vi "WriteConfig.vi"(8 "error in (no error)":errorcluster, 10 "Config":variant, 11 "RoomAlert in":refnum<class "RoomAlert.lvclass">) -> (0 "error out":errorcluster, 3 "RoomAlert out":refnum<class "RoomAlert.lvclass">)   [LabVIEW 2018, in "SensorPlugins.lvlib" / "RoomAlert.lvclass"]
doc: "Updates the configuration cluster."
uses:
  RoomAlert.lvclass
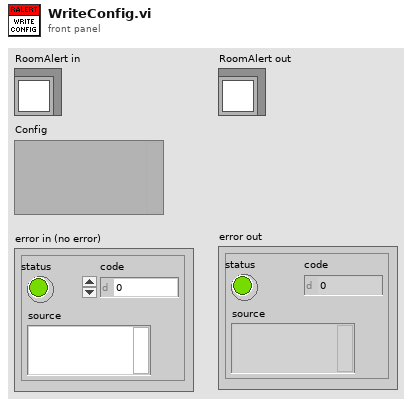
[diagram p1: front panel]
types:
  T1 = typedef "SensorPlugins.lvlib/RoomAlert.lvclass/MeasurementControls.ctl" = cluster{"Measurement RefreshTime (ms)":u32, "Measurement Name":string, "Timeout(ms)":i32, "Amber Warning Light Configuration":cluster{"Warning Temperture (Degrees C)":dbl, "Temperature Delta (Degrees C/Minute)":dbl, "Time Window (Minutes)":dbl}}
  T2 = typedef "SensorPlugins.lvlib/RoomAlert.lvclass/RoomAlertControls.ctl" = cluster{"Connected?":bool, "IP Address of SNMP Device":string, "Port (161)":u16, "Community Name":string, "Measurements To Read Array":u16[], "Update LightTower?":bool, "LightTower":cluster{"Red":bool, "Amber":bool, "Green":bool, "Audio":bool}, "RoomAlert Model ID":string, "Sensor OID Numbers":string[][], "Sensor Light Tower OID Numbers":string[][]}[]
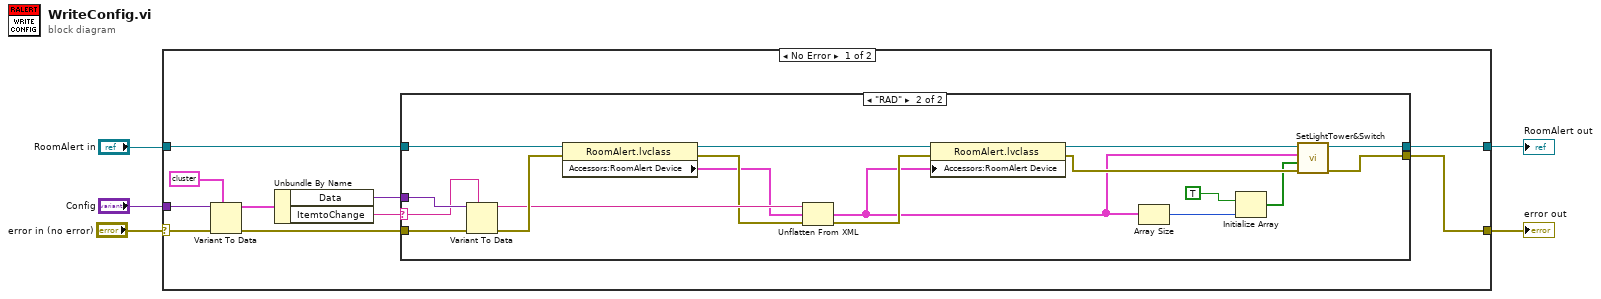
[diagram p0: block diagram]
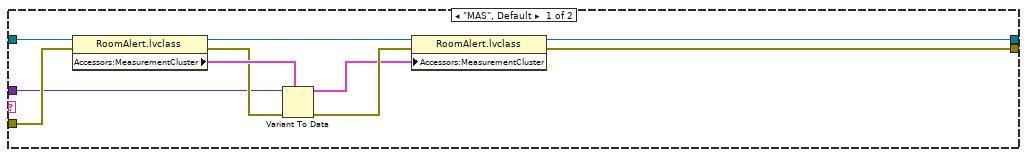
[diagram p2: hidden frame]
diagram:
  n1 = case shown="No Error" "error in (no error)" {
    selector: "error in (no error)" -> [w13 w45]
    tunnel: [w7 w45] -> w1
    tunnel: "RoomAlert in" -> [w15 w44]
    tunnel: [w6 w44] -> w2
    tunnel: "Config" -> [w14 _]
    frame No Error {
      n2 = Variant To Data(error in=w13, type=cluster{"Data":variant, "ItemtoChange":string} {"Data"=variant, "ItemtoChange"=""}, Variant=w14) -> (data=w10:cluster{"Data":variant, "ItemtoChange":string}, error out=w12:errorcluster)
      n3 = Unbundle By Name(w10) -> ("Data"=w9:variant, "ItemtoChange"=w8:string)
      n4 = case shown="\"RAD\"" w8 {
        selector: w8 -> [_ w38]
        tunnel: w15 -> [w25 w43]
        tunnel: [w23 w31] -> w6
        tunnel: [w22 w30] -> w7
        tunnel: w12 -> [w21 w40]
        tunnel: w9 -> [w18 w41]
        frame "MAS", Default {
          n5 = property class="RoomAlert.lvclass"(reference=w25, error in=w21) -> (reference out=w24:refnum<class "RoomAlert.lvclass">, error out=w19:errorcluster, "Accessors:MeasurementCluster"=w20:T1)
          n6 = Variant To Data(error in=w19, type=w20, Variant=w18) -> (data=w16:T1, error out=w17:errorcluster)
          n7 = property class="RoomAlert.lvclass"(reference=w24, error in=w17, "Accessors:MeasurementCluster"=w16) -> (reference out=w23:refnum<class "RoomAlert.lvclass">, error out=w22:errorcluster)
        }
        frame "RAD" {
          n8 = Variant To Data(error in=w40, type=w38, Variant=w41) -> (data=w37:string, error out=w39:errorcluster)
          n9 = property class="RoomAlert.lvclass"(reference=w43, error in=w39) -> (reference out=w42:refnum<class "RoomAlert.lvclass">, error out=w36:errorcluster, "Accessors:RoomAlert Device"=w35:T2)
          n10 = Unflatten From XML(xml string=w37, type=w35, error in (no error)=w36) -> (value=w29:T2, error out=w34:errorcluster)
          n11 = property class="RoomAlert.lvclass"(reference=w42, error in=w34, "Accessors:RoomAlert Device"=w29) -> (reference out=w33:refnum<class "RoomAlert.lvclass">, error out=w32:errorcluster)
          n12 = Array Size(array=w29) -> (size(s)=w28:i32)
          n13 = Initialize Array(TRUE, w28) -> (w26:bool[])
          n14 = call-dynamic "SetLightTower&Switch.vi"("error in (no error)"=w32, "UpdateValue? (F)"=w26, "RoomAlert Device"=w29, "RoomAlert in"=w33) -> ("error out"=w30:errorcluster, "RoomAlert out"=w31:refnum<class "RoomAlert.lvclass">)  [unwired: 6 in]
        }
      }
    }
    frame Error {
    }
  }
  "error out" <- w1
  "RoomAlert out" <- w2
